vi "Register for gRPC Server Events.vi"(8 "error in (no error)":errorcluster, 11 "CIFTemplatePlugin in":refnum<class "TemplatePlugin.lvclass">) -> (0 "error out":errorcluster, 2 "Event Registration Refnum":refnum<event-registration>, 3 "CIFTemplatePlugin out":refnum<class "TemplatePlugin.lvclass">)   [LabVIEW 2021, in "TemplatePlugin.lvclass"]
uses:
  TemplatePlugin.lvclass
  D:/dev/CIF-LVCore/src/CIFCore/Class/CIFCorePlugin.lvclass
  Grpc/Template_server/RPC Service/Template/Template.lvclass
  C:/Program Files/National Instruments/LabVIEW 2021/vi.lib/gRPC/LabVIEW gRPC Servicer/ServiceBase/ServiceBase.lvclass
  CIF-LVCore/src/CIFCore/Class/CIFCorePlugin.lvclass/CIFCorePlugin.ctl
  Grpc/Template_server/RPC Service/Template/Template.lvclass/Template.ctl
  CIF-LVCore/src/CIFCore/Common/Utilities/Add Error.vi
  <vilib>/CIF Foundation/CIF Utilities/Errors/Append Error Location.vi
  <vilib>/Utility/LVClass/Get LV Class Name.vi
  CIF-LVCore/src/CIFCore/Class/CIFCorePlugin.lvclass
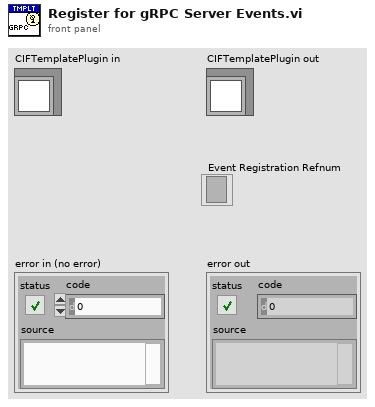
[diagram p1: front panel]
types:
  T1 = typedef "Template_server.lvlib/Template.lvclass/Server gRPC UEs.ctl" = cluster{"Template SetNumeric gRPC UE":refnum<user-event>, "Template GetResult gRPC UE":refnum<user-event>}
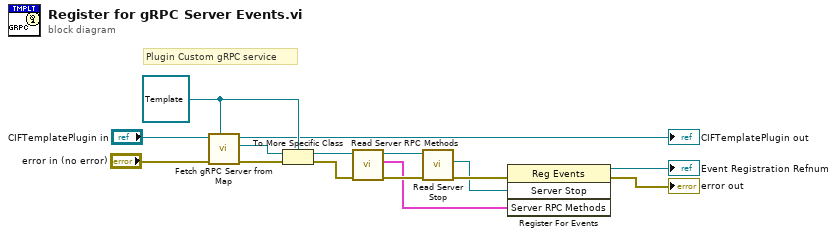
[diagram p0: block diagram]
diagram:
  w7 = refnum<class "Template.lvclass"> refnum ("CIFTemplatePlugin_server.lvlib:TemplatePlugin.lvclass")
  # "Plugin Custom gRPC service"
  n1 = call "Fetch gRPC Server from Map.vi"("gRPC Server Class type"=w7, "error in (no error)"="error in (no error)", "CIFCorePlugin in"="CIFTemplatePlugin in") -> ("error out"=w11:errorcluster, "gRPC Server Class out"=w10:refnum<class "ServiceBase.lvclass">, "CIFCorePlugin out"=→"CIFTemplatePlugin out":refnum<class "TemplatePlugin.lvclass">)  [unwired: 6 in]
  n2 = To More Specific Class(target class=w7, reference=w10, error in=w11) -> (specific class reference=w12:refnum<class "Template.lvclass">, error out=w6:errorcluster)
  n3 = call "Read Server RPC Methods.vi"("error in (no error)"=w6, "SignalGeneratorService in"=w12) -> ("error out"=w13:errorcluster, "Server RPC Methods"=w3:T1, "SignalGeneratorService out"=w14:refnum<class "Template.lvclass">)  [unwired: 7 in]
  n4 = call-dynamic "Read Server Stop.vi"("error in"=w13, "iService in"=w14) -> ("error out"=w4:errorcluster, "Server Stop"=w2:refnum<user-event>)  [unwired: 7 in, 1 out]
  n5 = register-events(error in=w4, w2, w3) -> (reference out=→"Event Registration Refnum":refnum<event-registration>, error out=→"error out":errorcluster)  [unwired: 1 in]
